vi "ProdaNG.Configurator.Popup.Add.vi"(6 "units simple":T3[](array[typedef]), 7 "Eleemnt Type":T1, 9 "Selected Element":T2, 10 "LastTS":T4) -> (1 "Selected elements value out":T2, 2 "Selected element out":T4, 4 "Reason out":string, 5 "OK?":bool)   [LabVIEW 2016]
uses:
  ProdaNG.Tree.Fglb.Data.ctl
  ProdaNG.Tree.Fglb.Element.ctl
  ProdaNG.Tree.Fglb.Value.ctl
  Controls/ProdaNG.UnitSimple.ctl
panel:
  in  "Unit":i32(ring) items=[""=0, "unknown"=-1, "%"=1, "bar"=2, "bar (abs)"=3, "mbar"=4, "bar/s"=5, "mbar/s"=6, "l/min"=7, "s"=8, "ms"=9, "mm"=10, "N"=11, "A"=12, "V"=13, "ohm"=14, "kohm"=15, "Hz"=16, "angle"=17, "count"=18, "bool"=19, "ASCII"=20, "Nm"=21, "kg"=22, "obr/min"=23, "ccm/min"=24, "mA"=25, "digit"=26, "us"=27, "stC"=28, "mBar/s"=29, "mA/s"=30, "undefined"=31, "WGrad"=32, "mH"=33, "-"=34, "tics"=35, "Nr"=36, "bar/min"=37, "us/mm"=38, "deg"=39, "mbar/deg"=40, "deg/s"=41]
  in  "Type":T5(ring)
  in  "Value2":dbl caption="High Limit" format="%.3f"
  in  "Value1":dbl caption="Low Limit / Param Value" format="%.3f"
  in  "Order":i32=1 min=1
  in  "Reason":string
  in  "Description":string
  in  "Button.Cancel":bool
  in  "Button.OK":bool
  out "Msg":string
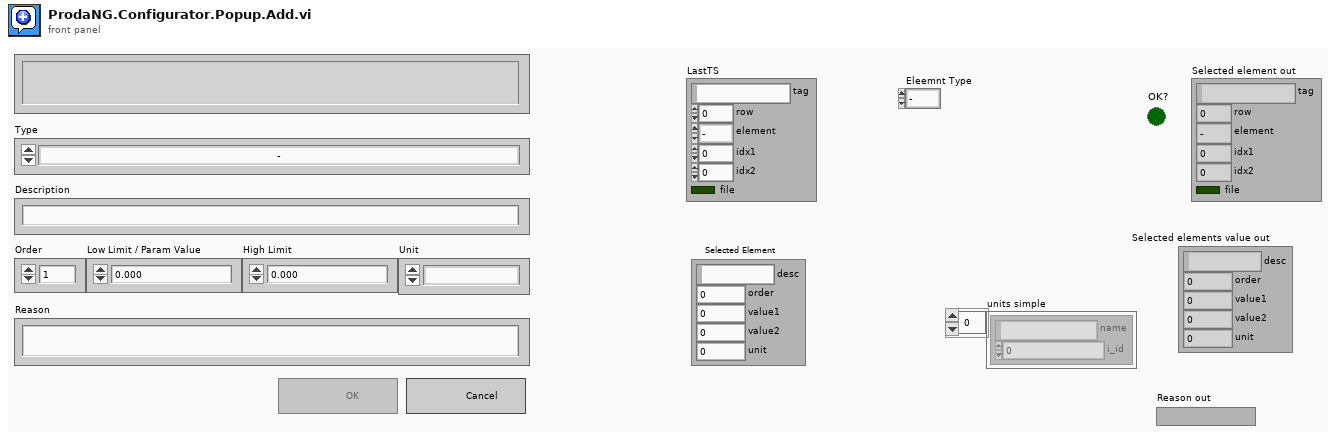
[diagram p1: front panel]
types:
  T1 = typedef "ProdaNG.Tree.Fglb.Element.ctl" = enum16{"-", "PP", "TS", "TP", "TV"}
  T2 = typedef "ProdaNG.Tree.Fglb.Value.ctl" = cluster{"desc":string, "order":i32, "value1":dbl, "value2":dbl, "unit":i32}
  T3 = typedef "ProdaNG.UnitSimple.ctl" = cluster{"name":string, "i_id":i32}
  T4 = typedef "ProdaNG.Tree.Fglb.Data.ctl" = cluster{"tag":string, "row":i32, "element":T1, "idx1":i32, "idx2":i32, "file":bool}
  T5 = enum16{"-", "Process Parameter", "Test Step", "Test Parameter", "Test Value"}
  T6 = enum8{"Enabled", "Disabled", "Disabled and Grayed Out"}
  T7 = typedef "LVStringsAndValuesArrayTypeDef_I32.ctl" = cluster{"String":string, "Value":i32}[]
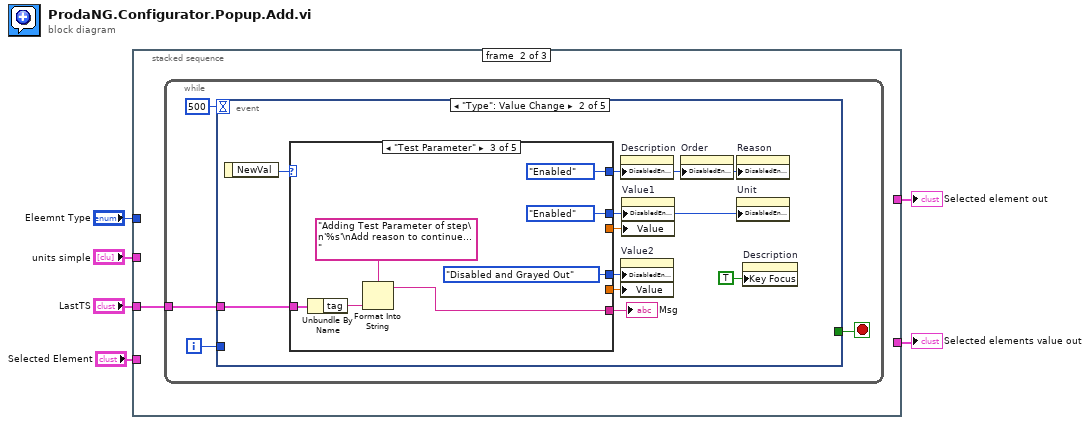
[diagram p0: block diagram]
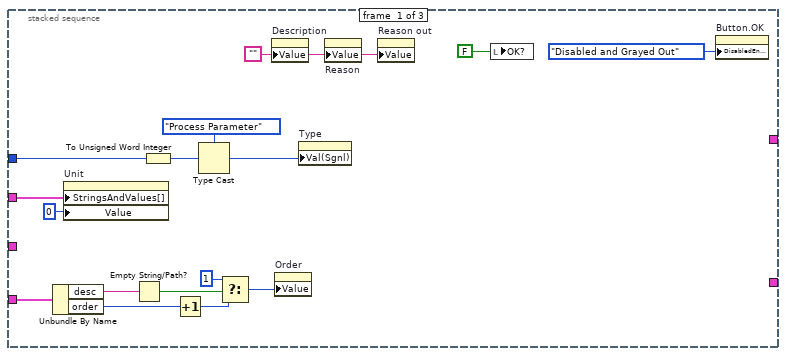
[diagram p2: hidden frame]
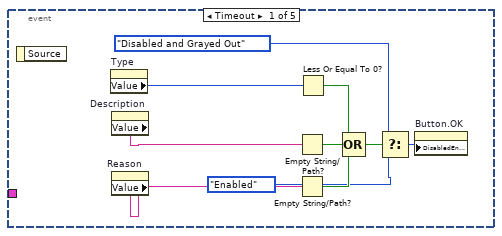
[diagram p3: hidden frame]
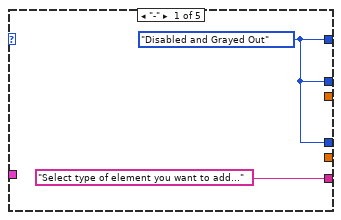
[diagram p4: hidden frame]
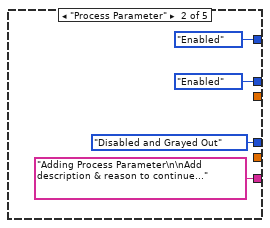
[diagram p5: hidden frame]
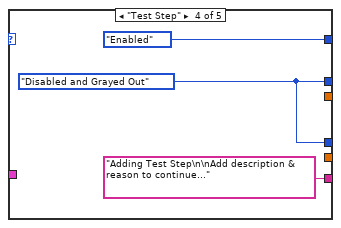
[diagram p6: hidden frame]
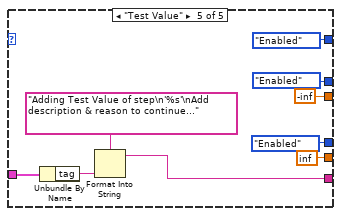
[diagram p7: hidden frame]
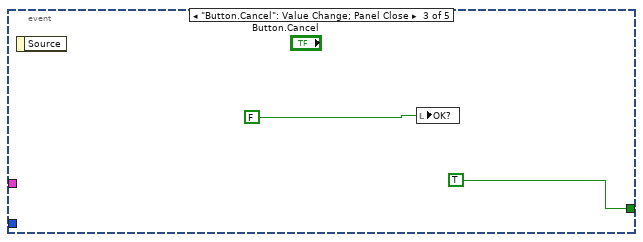
[diagram p8: hidden frame]
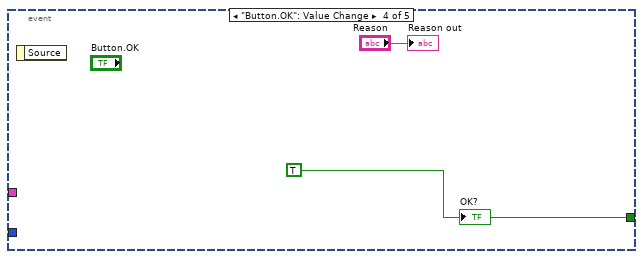
[diagram p9: hidden frame]
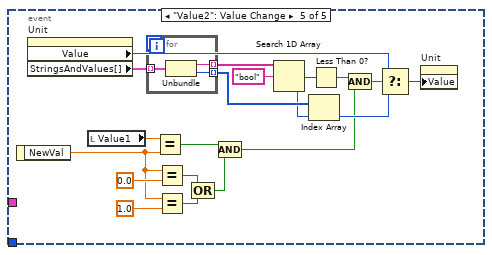
[diagram p10: hidden frame]
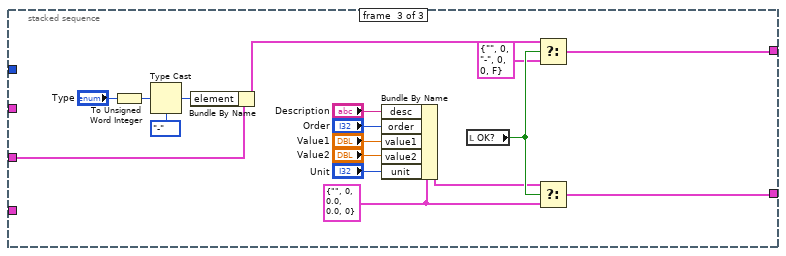
[diagram p11: hidden frame]
diagram:
  n1 = stacked-sequence {
    tunnel: [_ _ w114] -> w6
    tunnel: "LastTS" -> [_ w23 w112]
    tunnel: [_ _ w109] -> w4
    tunnel: "units simple" -> [w19 _ _]
    tunnel: "Selected Element" -> [w17 _ _]
    tunnel: "Eleemnt Type" -> [w7 _ _]
    frame #0 {
      w20 = ""
      n2 = Unbundle By Name(w17) -> ("desc"=w16:string, "order"=w13:i32)
      n3 = property on="Unit" class="Ring (strict)"("StringsAndValues[]"=w19, "Value"=0) -> ()  [unwired: 2 in, 2 out]
      n4 = Empty String/Path?(string/path=w16) -> (empty?=w15:bool)
      n5 = To Unsigned Word Integer(number=w7) -> (unsigned 16bit integer=w10:u16)
      n6 = Increment(x=w13) -> (x+1=w12:i32)
      n7 = Type Cast(type=T5."Process Parameter" ("Value (Signaling)"), x=w10) -> (*(type *) &x=w8:T5)
      n8 = Select(t=1 ("Order"), s=w15, f=w12) -> (s? t:f=w11:i32)
      n9 = property on="Description" class="Str"("Value"=w20) -> ()  [unwired: 2 in, 2 out]
      n10 = property on="Order" class="DigNum (strict)"("Value"=w11) -> ()  [unwired: 2 in, 2 out]
      n11 = property on="Type" class="Enum (strict)"("Val(Sgnl)"=w8) -> ()  [unwired: 2 in, 2 out]
      n12 = property on="Reason" class="Str"("Value"=w20) -> ()  [unwired: 2 in, 2 out]
      n13 = property on="Reason out" class="Str"("Value"=w20) -> ()  [unwired: 2 in, 2 out]
      n14 = local write "OK?"(FALSE ("OK?")) -> ()
      n15 = property on="Button.OK" class="Bool"("DisabledEnum"=T6."Disabled and Grayed Out" ("Disabled")) -> ()  [unwired: 2 in, 2 out]
    }
    frame #1 {
      n16 = while {
        tunnel: w23 -> [w24]
        i -> [w25]
        stop <- w27 stop-if-true
        n17 = event shown="[1] \"Type\": Value Change" {
          selector: _ -> [_ _ _ _ _]
          dyn-events: _ -> [_ _ _ _ _]
          timeout: 500 -> [_ _ _ _ _]
          tunnel: [_ _ TRUE ("OK?") w75 _] -> w27
          tunnel: w25 -> [_ _ _ _ _]
          tunnel: w24 -> [_ w41 _ _ _]
          event Timeout {
            n18 = event-data() -> ()  [unwired: 1 in, 1 out]
            n19 = property on="Type" class="Enum (strict)"() -> ("Value"=w33:T5)  [unwired: 2 in, 2 out]
            n20 = property on="Description" class="Str"() -> ("Value"=w31:string)  [unwired: 2 in, 2 out]
            n21 = property on="Reason" class="Str"() -> ("Value"=w32:string)  [unwired: 2 in, 2 out]
            n22 = Empty String/Path?(string/path=w31) -> (empty?=w34:bool)
            n23 = Empty String/Path?(string/path=w32) -> (empty?=w35:bool)
            n24 = Less Or Equal To 0?(x=w33) -> (x <= 0?=w36:bool)
            n25 = Compound Arithmetic op=OR(w36, w34, w35) -> (w37:bool)
            n26 = Select(t=T6."Disabled and Grayed Out" ("Disabled"), s=w37, f=T6."Enabled" ("Disabled")) -> (s? t:f=w28:T6)
            n27 = property on="Button.OK" class="Bool"("DisabledEnum"=w28) -> ()  [unwired: 2 in, 2 out]
          }
          event "Type": Value Change {
            n28 = event-data() -> ("NewVal"=w46:T5)  [unwired: 1 in]
            n29 = case shown="\"Test Parameter\"" w46 {
              tunnel: [w47 T6."Enabled" ("Disabled") T6."Enabled" ("Disabled") T6."Enabled" ("Disabled") T6."Enabled" ("Disabled")] -> w45
              tunnel: [w47 T6."Enabled" ("Disabled") T6."Enabled" ("Disabled") w61 T6."Enabled" ("Disabled")] -> w42
              tunnel: [_ _ _ _ -inf] -> w44
              tunnel: [_ _ _ _ inf] -> w43
              tunnel: w41 -> [_ _ w54 _ w66]
              tunnel: ["Select type of element you want to add..." ("format string") "Adding Process Parameter\n\nAdd description & reason to continue..." ("format string") w53 "Adding Test Step\n\nAdd description & reason to continue..." ("format string") w63] -> w40
              tunnel: [w47 T6."Disabled and Grayed Out" ("Disabled") T6."Disabled and Grayed Out" ("Disabled") w61 T6."Enabled" ("Disabled")] -> w39
              frame "-" {
                w47 = T6."Disabled and Grayed Out" ("Disabled")
              }
              frame "Process Parameter" {
              }
              frame "Test Parameter" {
                n30 = Unbundle By Name(w54) -> ("tag"=w56:string)
                n31 = Format Into String(format string="Adding Test Parameter of step\n'%s'\nAdd reason to continue...", w56) -> (resulting string=w53:string)  [unwired: 2 in, 1 out]
              }
              frame "Test Step" {
                w61 = T6."Disabled and Grayed Out" ("Disabled")
              }
              frame "Test Value" {
                n32 = Unbundle By Name(w66) -> ("tag"=w65:string)
                n33 = Format Into String(format string="Adding Test Value of step\n'%s'\nAdd description & reason to continue...", w65) -> (resulting string=w63:string)  [unwired: 2 in, 1 out]
              }
            }
            "Msg" <- w40
            n34 = property on="Description" class="Str"("DisabledEnum"=w45) -> ()  [unwired: 2 in, 2 out]
            n35 = property on="Value2" class="DigNum (strict)"("DisabledEnum"=w39, "Value"=w43) -> ()  [unwired: 2 in, 2 out]
            n36 = property on="Value1" class="DigNum (strict)"("DisabledEnum"=w42, "Value"=w44) -> ()  [unwired: 2 in, 2 out]
            n37 = property on="Order" class="DigNum (strict)"("DisabledEnum"=w45) -> ()  [unwired: 2 in, 2 out]
            n38 = property on="Reason" class="Str"("DisabledEnum"=w45) -> ()  [unwired: 2 in, 2 out]
            n39 = property on="Unit" class="Ring (strict)"("DisabledEnum"=w42) -> ()  [unwired: 2 in, 2 out]
            n40 = property on="Description" class="Str"("Key Focus"=TRUE) -> ()  [unwired: 2 in, 2 out]
          }
          event "Button.Cancel": Value Change; Panel Close {
            n41 = event-data() -> ()  [unwired: 1 in, 1 out]
            n42 = local write "OK?"(FALSE ("OK?")) -> ()
          }
          event "Button.OK": Value Change {
            w75 = TRUE ("OK?")
            n43 = event-data() -> ()  [unwired: 1 in, 1 out]
            "OK?" <- w75
            "Reason out" <- "Reason"
          }
          event "Value2": Value Change {
            n44 = event-data() -> ("NewVal"=w91:dbl)  [unwired: 1 in]
            n45 = property on="Unit" class="Ring (strict)"() -> ("Value"=w81:i32, "StringsAndValues[]"=w86:T7)  [unwired: 2 in, 2 out]
            n46 = local read "Value1"() -> (w94:dbl)
            n47 = for {
              tunnel: w86 -> [w97] mode=indexing
              tunnel: [w96] -> w85 mode=indexing
              tunnel: [w95] -> w83 mode=indexing
              n48 = Unbundle(w97) -> ("String"=w96:string, "Value"=w95:i32)
            }
            n49 = Equal?(x=w94, y=w91) -> (x = y?=w88:bool)
            n50 = Equal?(x=w91, y=0.0) -> (x = y?=w90:bool)
            n51 = Equal?(x=w91, y=1.0) -> (x = y?=w89:bool)
            n52 = Compound Arithmetic op=OR(w90, w89) -> (w87:bool)
            n53 = Compound Arithmetic op=AND(w88, w87) -> (w76:bool)
            n54 = Search 1D Array(1D array=w85, element="bool") -> (index of element=w82:i32)  [unwired: 1 in]
            n55 = Index Array(array=w83, index=w82) -> (element=w79:i32)
            n56 = Less Than 0?(x=w82) -> (x < 0?=w80:bool)
            n57 = Compound Arithmetic op=AND(w80, w76) -> (w77:bool)
            n58 = Select(t=w81, s=w77, f=w79) -> (s? t:f=w78:i32)
            n59 = property on="Unit" class="Ring (strict)"("Value"=w78) -> ()  [unwired: 2 in, 2 out]
          }
        }
      }
    }
    frame #2 {
      w98 = T2 {"desc"="", "order"=0, "value1"=0.0, "value2"=0.0, "unit"=0} ("Value")
      n60 = To Unsigned Word Integer(number="Type") -> (unsigned 16bit integer=w106:u16)
      n61 = Type Cast(type=ProdaNG.Tree.Fglb.Element."-" ("element"), x=w106) -> (*(type *) &x=w107:T1)
      n62 = Bundle By Name(cluster=w112, "element"=w107) -> (w111:T4)
      n63 = Bundle By Name(cluster=w98, "desc"="Description", "order"="Order", "value1"="Value1", "value2"="Value2", "unit"="Unit") -> (w100:T2)
      n64 = local read "OK?"() -> (w113:bool)
      n65 = Select(t=w111, s=w113, f=T4 {"tag"="", "row"=0, "element"=enum."-", "idx1"=0, "idx2"=0, "file"=FALSE}) -> (s? t:f=w109:T4)
      n66 = Select(t=w100, s=w113, f=w98) -> (s? t:f=w114:T2)
    }
  }
  "Selected elements value out" <- w6
  "Selected element out" <- w4
